vi "CODMn停止命令 (子VI).vi"   [LabVIEW 2016, in "斯坦道CODMn.lvlib"]
uses:
  <vilib>/Plasmionique/MB Master/MB_Master_Serial/MB_Master_Serial.lvclass
  D:/Program Files (x86)/National Instruments/LabVIEW 2016/vi.lib/Plasmionique/MB Master/MB_Master/MB_Master.lvclass
  <vilib>/Plasmionique/MB Master/MB Master.lvlib
types:
  T1 = cluster{"baud rate (bps)":u32, "stop bits":u16, "parity":u16, "flow control":u16, "timeout":u32, "retries":i32}
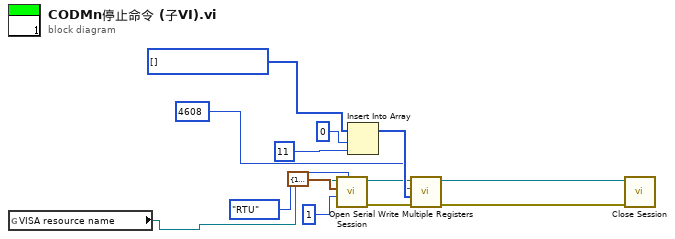
[diagram p0: block diagram]
diagram:
  n1 = global read "COD浓度全局变量.vi" "VISA resource name"() -> (w1:refnum<visa-resource-name>)
  n2 = call <vilib>:"Open Serial Session.vi"("Mode (RTU)"=enum16{"RTU", "ASCII"}."RTU", "Slave ID"=u8 1, "Serial Config"=T1 {"baud rate (bps)"=115200, "stop bits"=10, "parity"=0, "flow control"=0, "timeout"=1000, "retries"=1}, "VISA Resource"=w1) -> ("Error out"=w13:errorcluster, "MB_Serial session"=w4:refnum<class "MB_Master_Serial.lvclass">)  [unwired: 6 in]
  n3 = Insert Into Array(array=u16[] [] ("values"), index=0 ("索引"), new element=u16 11 ("address")) -> (w12:u16[])
  n4 = call <vilib>:"Write Multiple Registers.vi"("error in (no error)"=w13, "values"=w12, "starting address"=u16 4608 ("address"), "MB session in"=w4) -> ("error out"=w2:errorcluster, "MB session out"=w3:refnum<class "MB_Master_Serial.lvclass">)  [unwired: 6 in]
  n5 = call-dynamic "Close Session.vi"("error in (no error)"=w2, "MB_Serial session"=w3) -> ()  [unwired: 9 in, 1 out]
